vi "Find Top Level VI.vi"(8 "Error In":errorcluster, 11 "Panel Helper in":refnum<class "Panel Helper.lvclass">) -> (0 "Error Out":errorcluster, 1 "Found?":bool, 2 "Top Level Panel":string)   [LabVIEW 2017, in "MGI-Panel Manager.lvlib" / "Panel Helper.lvclass"]
doc: "Tries to find the panel associated with the top-level VI for the caller.\n----\nPlease see the following web address for additional documentation and tutorial information:\nhttp://www.mooregoodideas.com/mgi-panel-manager/\n\nAuthor: Derek Trepanier\n\nCopyright (c) 2018, Moore Good Ideas, Inc.\n\nAll rights reserved.\n\nRedistribution and use in source and binary forms, with or without modification, are permitted provided that the following conditions are met:\n\n * Redistributions of source code must retain the above copyright notice, this list of conditions and the following disclaimer.\n * Redistributions in binary form must reproduce the above copyright notice, this list of conditions and the following disclaimer in the documentation and/or other materials provided with the distribution.\n * Neither the name of Moore Good Ideas, Inc. nor the names of its contributors may be used to endorse or promote products derived from this software without specific prior written permission.\n\nTHIS SOFTWARE IS PROVIDED BY THE COPYRIGHT HOLDERS AND CONTRIBUTORS \"AS IS\" AND ANY EXPRESS OR IMPLIED WARRANTIES, INCLUDING, BUT NOT LIMITED TO, THE IMPLIED WARRANTIES OF MERCHANTABILITY AND FITNESS FOR A PARTICULAR PURPOSE ARE DISCLAIMED. IN NO EVENT SHALL THE COPYRIGHT OWNER OR CONTRIBUTORS BE LIABLE FOR ANY DIRECT, INDIRECT, INCIDENTAL, SPECIAL, EXEMPLARY, OR CONSEQUENTIAL DAMAGES (INCLUDING, BUT NOT LIMITED TO, PROCUREMENT OF SUBSTITUTE GOODS OR SERVICES; LOSS OF USE, DATA, OR PROFITS; OR BUSINESS INTERRUPTION) HOWEVER CAUSED AND ON ANY THEORY OF LIABILITY, WHETHER IN CONTRACT, STRICT LIABILITY, OR TORT (INCLUDING NEGLIGENCE OR OTHERWISE) ARISING IN ANY WAY OUT OF THE USE OF THIS SOFTWARE, EVEN IF ADVISED OF THE POSSIBILITY OF SUCH DAMAGE."
uses:
  Panel Helper.lvclass
  Panel Helper.lvclass/Panel Helper.ctl
  Panel/Panel.lvclass
  MGI-Panel Manager.lvlib
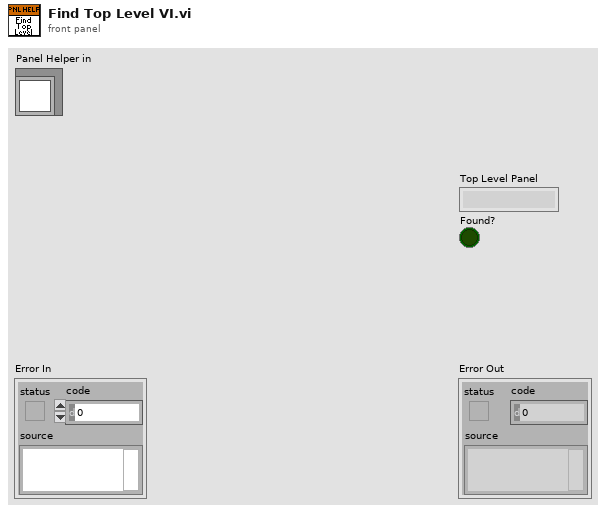
[diagram p1: front panel]
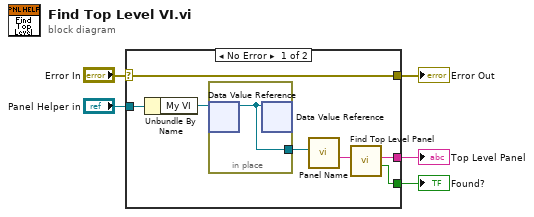
[diagram p0: block diagram]
diagram:
  n1 = case shown="No Error" "Error In" {
    selector: "Error In" -> [w12 w14]
    tunnel: [w12 w14] -> w4
    tunnel: "Panel Helper in" -> [w11 _]
    tunnel: [w10 _] -> w2
    tunnel: [w9 _] -> w1
    frame No Error {
      n2 = Unbundle By Name(w11) -> ("My VI"=w8:refnum<data-value>)
      n3 = in-place {
        in-place-border: [w13] -> w7
        n4 = in-place-dvr #1(w8) -> (w13:refnum<vi>)  [unwired: 1 out]
        n5 = in-place-dvr #1(w13) -> ()  [unwired: 2 out]
      }
      n6 = call "Panel Name.vi"("VI in"=w7) -> ("Name"=w6:string)  [unwired: 9 in, 1 out]
      n7 = call "Find Top Level Panel.vi"("VI (Caller)"=w6) -> ("Found?"=w9:bool, "Top Level Panel"=w10:string)  [unwired: 9 in]
    }
    frame Error {
    }
  }
  "Error Out" <- w4
  "Top Level Panel" <- w2
  "Found?" <- w1
